vi "Replicate.vi"(0 "msgrM":T1, 1 "subchannel":i32) -> (2 "msgrM0":T1)   [LabVIEW 2019, in "MessengerM.lvlib"]
uses:
  MessengerM.lvlib
  ))Channel.ctl
  Element.ctl
  Endpoint.vi
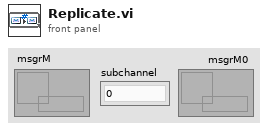
[diagram p1: front panel]
types:
  T1 = typedef "MessengerM.lvlib/))Channel.ctl" = refnum<queue>
  T2 = typedef "MessengerM.lvlib/Element.ctl" = string
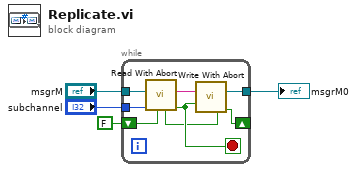
[diagram p0: block diagram]
diagram:
  n1 = while {
    tunnel: "msgrM" -> [w8]
    tunnel: "subchannel" -> [w12]
    tunnel: [w10] -> w3
    shift-right: [w7] -> _
    shift-left: FALSE ("aborted?") -> [w6]
    stop <- w11 stop-if-true
    n2 = call "Read With Abort.vi"("abort (F)"=w6, "subchannel (0)"=w12, "channel"=w8) -> ("last element?"=w11:bool, "element"=w9:T2, "aborted?"=w5:bool)  [unwired: 3 in, 3 out]
    n3 = call "Write With Abort.vi"("element"=w9, "last element? (F)"=w11, "abort (F)"=w5) -> ("channel"=w10:T1, "aborted?"=w7:bool)  [unwired: 8 in, 3 out]
  }
  "msgrM0" <- w3
